vi "ErrorWindowTest.vi"(0 "Connection ID TB":refnum<k5>, 1 "connection ID CC":refnum<k5>, 2 "IP ADDRESS":string="192.168.0.100", 3 "IP ADDRESS 2":string="192.168.0.100", 4 "error in (no error)":errorcluster) -> (5 "REPORT LOG":string, 6 "PASS / FAIL":bool, 7 "error out":errorcluster)   [LabVIEW 2013]
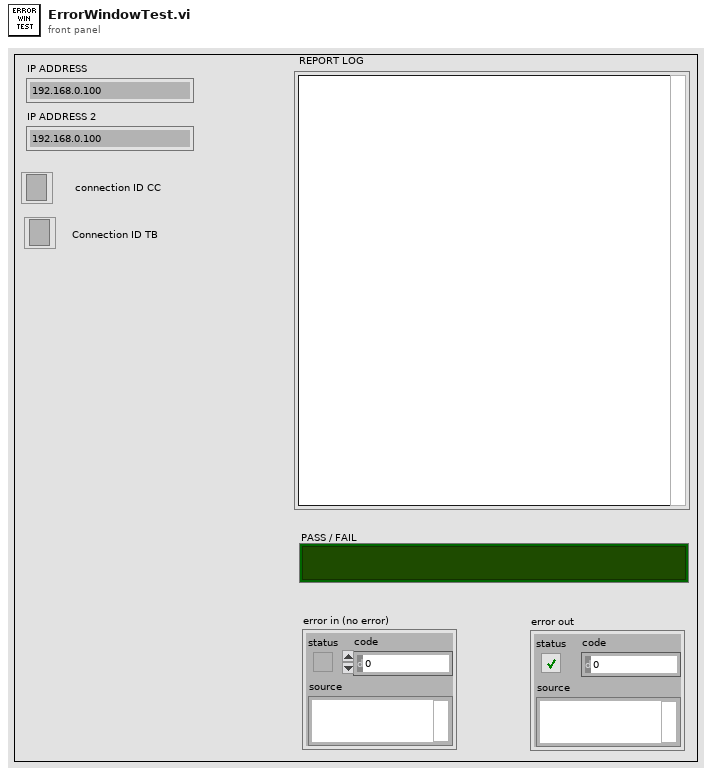
[diagram p1: front panel]
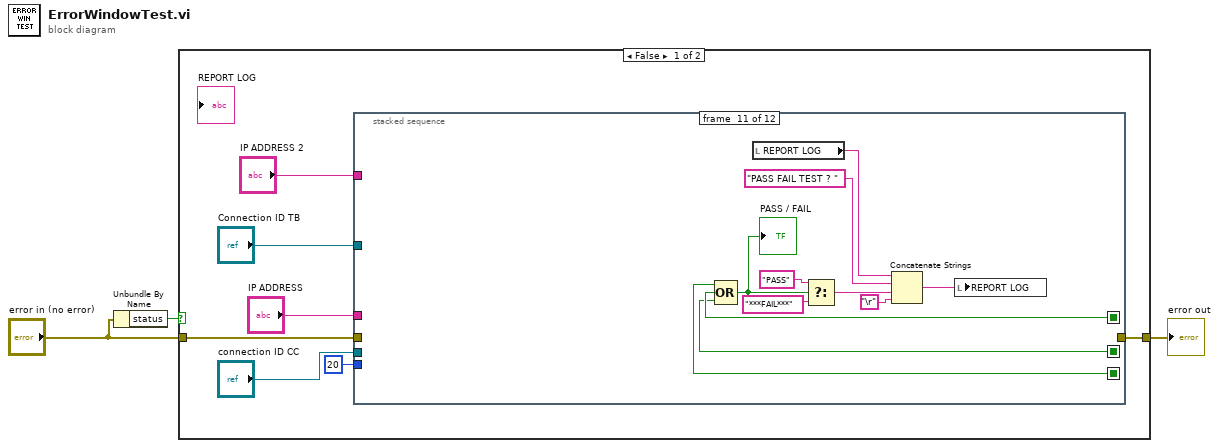
[diagram p0: block diagram]
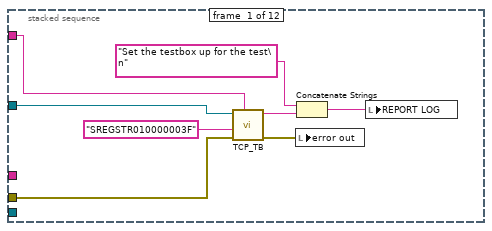
[diagram p2: hidden frame]
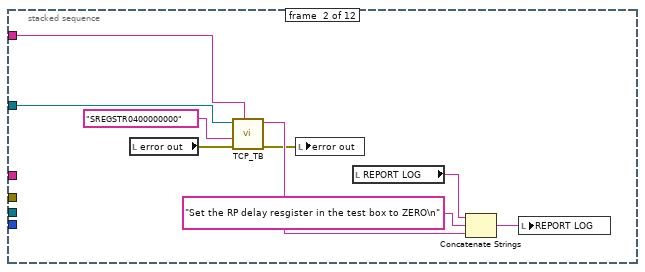
[diagram p3: hidden frame]
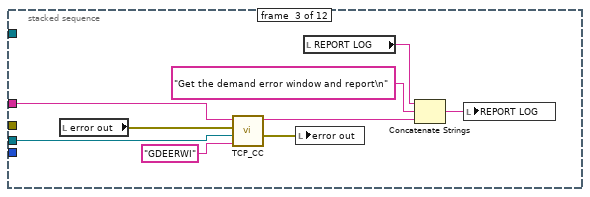
[diagram p4: hidden frame]
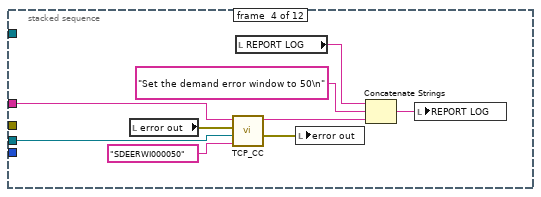
[diagram p5: hidden frame]
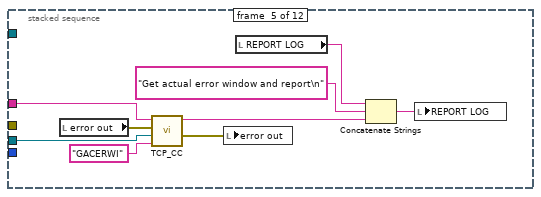
[diagram p6: hidden frame]
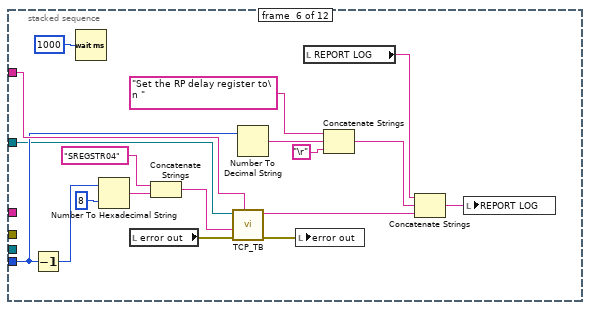
[diagram p7: hidden frame]
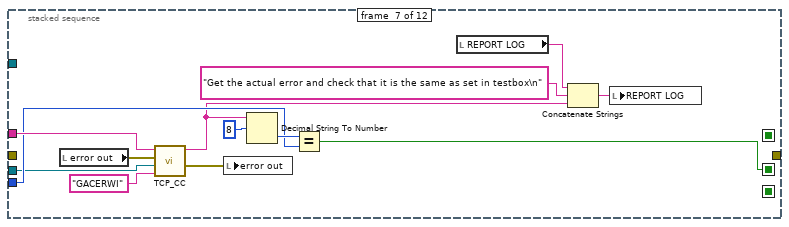
[diagram p8: hidden frame]
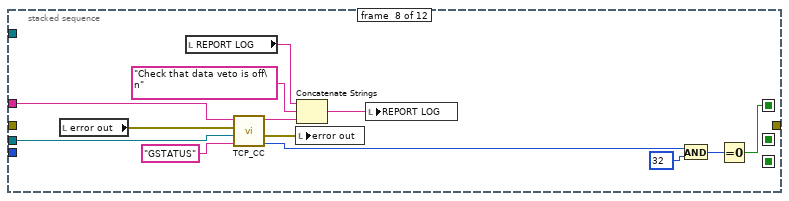
[diagram p9: hidden frame]
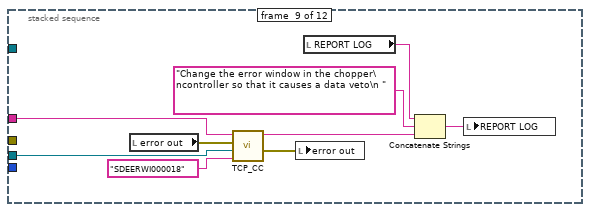
[diagram p10: hidden frame]
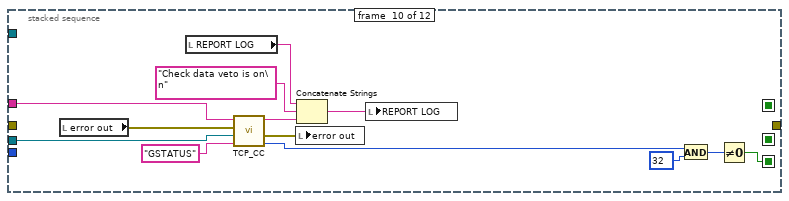
[diagram p11: hidden frame]
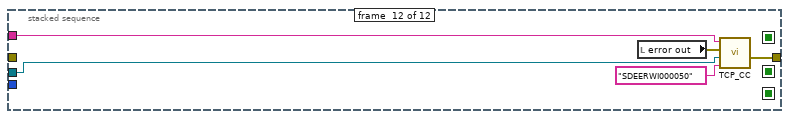
[diagram p12: hidden frame]
diagram:
  n1 = Unbundle By Name("error in (no error)") -> ("status"=w3:bool)
  n2 = case shown="False" w3 {
    tunnel: "error in (no error)" -> [w4 w137]
    tunnel: [w5 w137] -> w1
    frame False {
      n3 = stacked-sequence {
        seq-local: [_ _ _ _ _ _ _ _ _ w111 _ _] -> [_ _ _ _ _ _ _ _ _ _ w128 _]
        seq-local: [_ _ _ _ _ _ _ w89 _ _ _ _] -> [_ _ _ _ _ _ _ _ _ _ w127 _]
        seq-local: [_ _ _ _ _ _ w76 _ _ _ _ _] -> [_ _ _ _ _ _ _ _ _ _ w126 _]
        tunnel: "IP ADDRESS" -> [_ _ w36 w45 w54 _ w85 w98 w107 w120 _ w136]
        tunnel: "IP ADDRESS 2" -> [w18 w27 _ _ _ w72 _ _ _ _ _ _]
        tunnel: 20 -> [_ _ _ _ _ w64 w81 _ _ _ _ _]
        tunnel: "connection ID CC" -> [_ _ w30 w39 w48 _ w75 w88 w101 w110 _ w134]
        tunnel: "Connection ID TB" -> [w13 w21 _ _ _ w57 _ _ _ _ _ _]
        tunnel: [_ _ _ _ _ _ _ _ _ _ _ w133] -> w5
        tunnel: w4 -> [w12 _ _ _ _ _ _ _ _ _ _ _]
        frame #0 {
          n4 = call "TCP_TB.vi"("IP ADDRESS"=w18, "error in (no error)"=w12, "COMMAND"="SREGSTR010000003F", "Connection ID IN"=w13) -> ("error out"=w11:errorcluster, "Their Response:"=w15:string)  [unwired: 2 in, 1 out]
          n5 = local write "error out"(w11) -> ()
          n6 = Concatenate Strings("Set the testbox up for the test\n" ("COMMAND"), w15) -> (w14:string)
          n7 = local write "REPORT LOG"(w14) -> ()
        }
        frame #1 {
          n8 = local read "error out"() -> (w19:errorcluster)
          n9 = call "TCP_TB.vi"("IP ADDRESS"=w27, "error in (no error)"=w19, "COMMAND"="SREGSTR0400000000", "Connection ID IN"=w21) -> ("error out"=w20:errorcluster, "Their Response:"=w22:string)  [unwired: 2 in, 1 out]
          n10 = local write "error out"(w20) -> ()
          n11 = local read "REPORT LOG"() -> (w25:string)
          n12 = Concatenate Strings(w25, "Set the RP delay resgister in the test box to ZERO\n" ("COMMAND"), w22) -> (w24:string)
          n13 = local write "REPORT LOG"(w24) -> ()
        }
        frame #2 {
          n14 = local read "error out"() -> (w29:errorcluster)
          n15 = call "TCP_CC.vi"("COMMAND"="GDEERWI", "connection ID"=w30, "error in (no error)"=w29, "IP ADDRESS"=w36) -> ("error out"=w28:errorcluster, "The Response:"=w31:string)  [unwired: 2 out]
          n16 = local write "error out"(w28) -> ()
          n17 = local read "REPORT LOG"() -> (w34:string)
          n18 = Concatenate Strings(w34, "Get the demand error window and report\n" ("COMMAND"), w31) -> (w33:string)
          n19 = local write "REPORT LOG"(w33) -> ()
        }
        frame #3 {
          n20 = local read "error out"() -> (w38:errorcluster)
          n21 = call "TCP_CC.vi"("COMMAND"="SDEERWI000050", "connection ID"=w39, "error in (no error)"=w38, "IP ADDRESS"=w45) -> ("error out"=w37:errorcluster, "The Response:"=w40:string)  [unwired: 2 out]
          n22 = local read "REPORT LOG"() -> (w43:string)
          n23 = local write "error out"(w37) -> ()
          n24 = Concatenate Strings(w43, "Set the demand error window to 50\n" ("COMMAND"), w40) -> (w42:string)
          n25 = local write "REPORT LOG"(w42) -> ()
        }
        frame #4 {
          n26 = local read "error out"() -> (w47:errorcluster)
          n27 = call "TCP_CC.vi"("COMMAND"="GACERWI", "connection ID"=w48, "error in (no error)"=w47, "IP ADDRESS"=w54) -> ("error out"=w46:errorcluster, "The Response:"=w49:string)  [unwired: 2 out]
          n28 = local write "error out"(w46) -> ()
          n29 = local read "REPORT LOG"() -> (w52:string)
          n30 = Concatenate Strings(w52, "Get actual error window and report\n" ("COMMAND"), w49) -> (w51:string)
          n31 = local write "REPORT LOG"(w51) -> ()
        }
        frame #5 {
          n32 = Decrement(x=w64) -> (x-1=w70:i32)
          n33 = Wait (ms)(milliseconds to wait=u32 1000) -> ()  [unwired: 1 out]
          n34 = Number To Hexadecimal String(1:i16 8 ("width (-)"), 2:w70) -> (0:w67:string)
          n35 = local read "error out"() -> (w56:errorcluster)
          n36 = Concatenate Strings("SREGSTR04" ("COMMAND"), w67) -> (w66:string)
          n37 = call "TCP_TB.vi"("IP ADDRESS"=w72, "error in (no error)"=w56, "COMMAND"=w66, "Connection ID IN"=w57) -> ("error out"=w55:errorcluster, "Their Response:"=w58:string)  [unwired: 2 in, 1 out]
          n38 = Number To Decimal String(number=w64) -> (decimal integer string=w63:string)  [unwired: 1 in]
          n39 = local write "error out"(w55) -> ()
          n40 = local read "REPORT LOG"() -> (w61:string)
          n41 = Concatenate Strings("Set the RP delay register to\n " ("COMMAND"), w63, "\r") -> (w59:string)
          n42 = Concatenate Strings(w61, w59, w58) -> (w60:string)
          n43 = local write "REPORT LOG"(w60) -> ()
        }
        frame #6 {
          n44 = local read "error out"() -> (w74:errorcluster)
          n45 = call "TCP_CC.vi"("COMMAND"="GACERWI", "connection ID"=w75, "error in (no error)"=w74, "IP ADDRESS"=w85) -> ("error out"=w73:errorcluster, "The Response:"=w77:string)  [unwired: 2 out]
          n46 = local write "error out"(w73) -> ()
          n47 = Decimal String To Number(string=w77, offset=8) -> (number=w82:i32)  [unwired: 1 in, 1 out]
          n48 = Equal?(x=w82, y=w81) -> (x = y?=w76:bool)
          n49 = local read "REPORT LOG"() -> (w80:string)
          n50 = Concatenate Strings(w80, "Get the actual error and check that it is the same as set in testbox\n" ("COMMAND"), w77) -> (w79:string)
          n51 = local write "REPORT LOG"(w79) -> ()
        }
        frame #7 {
          n52 = local read "error out"() -> (w87:errorcluster)
          n53 = local read "REPORT LOG"() -> (w93:string)
          n54 = call "TCP_CC.vi"("COMMAND"="GSTATUS", "connection ID"=w88, "error in (no error)"=w87, "IP ADDRESS"=w98) -> ("number"=w96:u32, "error out"=w86:errorcluster, "The Response:"=w90:string)  [unwired: 1 out]
          n55 = local write "error out"(w86) -> ()
          n56 = Concatenate Strings(w93, "Check that data veto is off\n" ("COMMAND"), w90) -> (w92:string)
          n57 = local write "REPORT LOG"(w92) -> ()
          n58 = And(x=w96, y=u32 32) -> (x .and. y?=w94:u32)
          n59 = Equal To 0?(x=w94) -> (x = 0?=w89:bool)
        }
        frame #8 {
          n60 = local read "error out"() -> (w100:errorcluster)
          n61 = call "TCP_CC.vi"("COMMAND"="SDEERWI000018", "connection ID"=w101, "error in (no error)"=w100, "IP ADDRESS"=w107) -> ("error out"=w99:errorcluster, "The Response:"=w102:string)  [unwired: 2 out]
          n62 = local write "error out"(w99) -> ()
          n63 = local read "REPORT LOG"() -> (w105:string)
          n64 = Concatenate Strings(w105, "Change the error window in the chopper\ncontroller so that it causes a data veto\n " ("COMMAND"), w102) -> (w104:string)
          n65 = local write "REPORT LOG"(w104) -> ()
        }
        frame #9 {
          n66 = local read "error out"() -> (w109:errorcluster)
          n67 = local read "REPORT LOG"() -> (w115:string)
          n68 = call "TCP_CC.vi"("COMMAND"="GSTATUS", "connection ID"=w110, "error in (no error)"=w109, "IP ADDRESS"=w120) -> ("number"=w118:u32, "error out"=w108:errorcluster, "The Response:"=w112:string)  [unwired: 1 out]
          n69 = local write "error out"(w108) -> ()
          n70 = Concatenate Strings(w115, "Check data veto is on\n" ("COMMAND"), w112) -> (w114:string)
          n71 = local write "REPORT LOG"(w114) -> ()
          n72 = And(x=w118, y=u32 32) -> (x .and. y?=w116:u32)
          n73 = Not Equal To 0?(x=w116) -> (x != 0?=w111:bool)
        }
        frame #10 {
          n74 = Compound Arithmetic op=OR(w128, w127, w126) -> (w124:bool)
          "PASS / FAIL" <- w124
          n75 = local read "REPORT LOG"() -> (w131:string)
          n76 = Select(t="PASS" ("COMMAND"), s=w124, f="***FAIL***" ("COMMAND")) -> (s? t:f=w121:string)
          n77 = Concatenate Strings(w131, "PASS FAIL TEST ? " ("COMMAND"), w121, "\r") -> (w130:string)
          n78 = local write "REPORT LOG"(w130) -> ()
        }
        frame #11 {
          n79 = local read "error out"() -> (w132:errorcluster)
          n80 = call "TCP_CC.vi"("COMMAND"="SDEERWI000050", "connection ID"=w134, "error in (no error)"=w132, "IP ADDRESS"=w136) -> ("error out"=w133:errorcluster)  [unwired: 3 out]
        }
      }
    }
    frame True {
    }
  }
  "error out" <- w1
